vi "Connect.vi"(8 "error in (no error)":errorcluster, 11 "NI-DAQ in":refnum<class "NI-DAQ.lvclass">) -> (0 "error out":errorcluster, 3 "NI-DAQ out":refnum<class "NI-DAQ.lvclass">)   [LabVIEW 2016, in "NI-DAQ.lvclass"]
uses:
  NI-DAQ.lvclass
  NI-DAQ.lvclass/NI-DAQ.ctl
  I-O Folder/I-O.lvclass
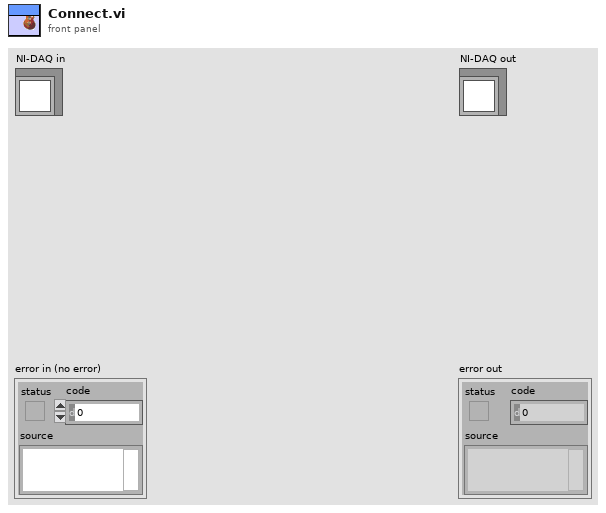
[diagram p1: front panel]
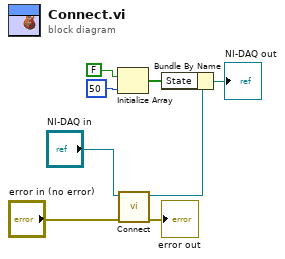
[diagram p0: block diagram]
diagram:
  n1 = Initialize Array(FALSE, 50 ("dimension size")) -> (w3:bool[])
  n2 = call-parent "Connect.vi"("error in (no error)"="error in (no error)", "I-O in"="NI-DAQ in") -> ("error out"=→"error out":errorcluster, "I-O out"=w2:refnum<class "NI-DAQ.lvclass">)  [unwired: 8 in]
  n3 = Bundle By Name(cluster=w2, "State"=w3) -> (→"NI-DAQ out":refnum<class "NI-DAQ.lvclass">)
